vi "write_params.vi"(8 "error in (no error)":errorcluster, 10 "params":T1={"solver"="svd", "shrinkage"={"shrinkage_type"="None", "shrinkage_float"=0.0}, "priors"={"priors_type"="None", "priors_list"=[]}, "n_components"={"n_components_type"="None", "n_components_int"=0.0}, "store_covariance"=FALSE, "tol"=0.0001}, 11 "LinearDiscriminantAnalysis in":refnum<class "LinearDiscriminantAnalysis.lvclass">) -> (0 "error out":errorcluster, 3 "LinearDiscriminantAnalysis out":refnum<class "LinearDiscriminantAnalysis.lvclass">)   [LabVIEW 2020, in "LinearDiscriminantAnalysis.lvclass"]
uses:
  LinearDiscriminantAnalysis.lvclass
  Controls/linear_discriminant_analysis_params.ctl
  LinearDiscriminantAnalysis.lvclass/LinearDiscriminantAnalysis.ctl
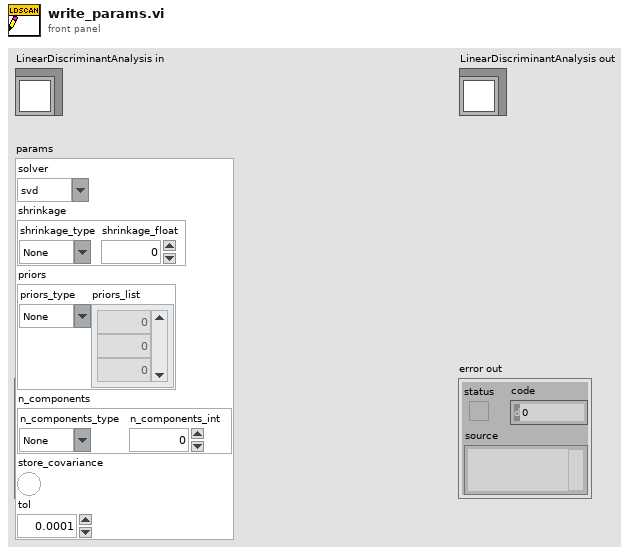
[diagram p1: front panel]
types:
  T1 = typedef "linear_discriminant_analysis_params.ctl" = cluster{"solver":string, "shrinkage":cluster{"shrinkage_type":string, "shrinkage_float":dbl}, "priors":cluster{"priors_type":string, "priors_list":dbl[]}, "n_components":cluster{"n_components_type":string, "n_components_int":dbl}, "store_covariance":bool, "tol":dbl}
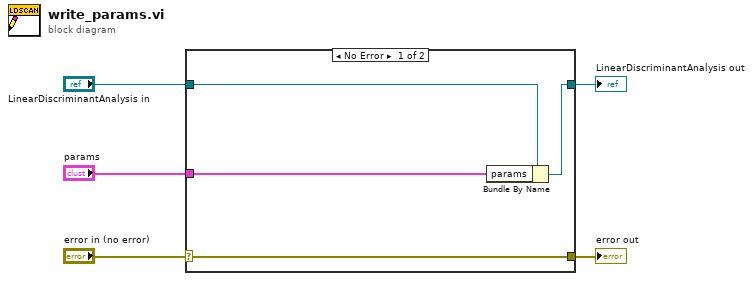
[diagram p0: block diagram]
diagram:
  n1 = case shown="No Error" "error in (no error)" {
    selector: "error in (no error)" -> [w9 w10]
    tunnel: [w9 w10] -> w4
    tunnel: [w7 w11] -> w2
    tunnel: "LinearDiscriminantAnalysis in" -> [w8 w11]
    tunnel: "params" -> [w6 _]
    frame No Error {
      n2 = Bundle By Name(cluster=w8, "params"=w6) -> (w7:refnum<class "LinearDiscriminantAnalysis.lvclass">)
    }
    frame Error {
    }
  }
  "error out" <- w4
  "LinearDiscriminantAnalysis out" <- w2
